vi "Drive Straight 2.vi"(9 "Time":dbl, 10 "Angle":dbl, 11 "RobotDriveDevRef in":T1) -> (3 "RobotDriveDevRef out":T1)   [LabVIEW 2015]
uses:
  <vilib>/Rock Robotics/WPI/RobotDrive/WPI_RobotDriveDevRef.ctl
  <vilib>/Rock Robotics/WPI/MotorControl/WPI_MotorControlDeviceRef.ctl
  <vilib>/Rock Robotics/WPI/MotorControl/WPI_MotorControlType.ctl
  <vilib>/Rock Robotics/SystemInterfaces/DIO/FPGA_DIOPWMChannel.ctl
  <vilib>/Rock Robotics/WPI/PWM/WPI_PWMDeadband.ctl
  <vilib>/Rock Robotics/WPI/CAN/Jaguar/SubVIs/WPI_CANJaguar_ControlMode.ctl
  <vilib>/Rock Robotics/WPI/CAN/TalonSRX/WPI_CANTalonSRX_APIControlMode.ctl
  <vilib>/Rock Robotics/Network Tables/NT Read Number.vi
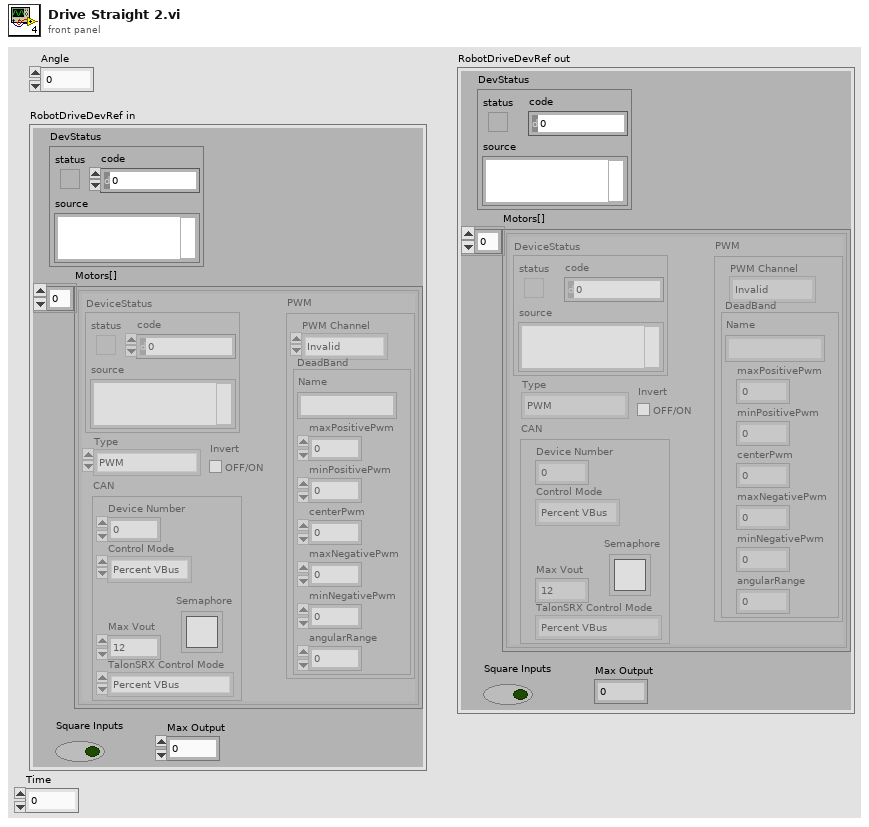
[diagram p1: front panel]
types:
  T1 = typedef "WPI_RobotDriveDevRef.ctl" = cluster{"DevStatus":errorcluster, "Motors[]":T2[], "Square Inputs":bool, "Max Output":dbl}
  T2 = typedef "WPI_MotorControlDeviceRef.ctl" = cluster{"DeviceStatus":errorcluster, "Type":T3, "PWM":cluster{"PWM Channel":T4, "DeadBand":T5}, "CAN":cluster{"Device Number":u8, "Control Mode":T6, "Semaphore":T7, "Max Vout":dbl, "TalonSRX Control Mode":T8}, "Invert":bool}
  T3 = typedef "WPI_MotorControlType.ctl" = enum16{"PWM", "CAN", "CANTalonSRX"}
  T4 = typedef "FPGA_DIOPWMChannel.ctl" = enum8{"PWM 0", "PWM 1", "PWM 2", "PWM 3", "PWM 4", "PWM 5", "PWM 6", "PWM 7", "PWM 8", "PWM 9", "PWM MXP 0", "PWM MXP 1", "PWM MXP 2", "PWM MXP 3", "PWM MXP 4", "PWM MXP 5", "PWM MXP 6", "PWM MXP 7", "PWM MXP 8", "PWM MXP 9", "Invalid"}
  T5 = typedef "WPI_PWMDeadband.ctl" = cluster{"Name":string, "maxPositivePwm":i32, "minPositivePwm":i32, "centerPwm":i32, "maxNegativePwm":i32, "minNegativePwm":i32, "angularRange":u16}
  T6 = typedef "WPI_CANJaguar_ControlMode.ctl" = enum8{"Percent VBus", "Current", "Speed", "Position", "Voltage"}
  T7 = typedef "Semaphore RefNum" = refnum<k1>
  T8 = typedef "WPI_CANTalonSRX_APIControlMode.ctl" = enum8{"Percent VBus", "Speed", "Position", "Slave", "Unchanged / Invalid", "Voltage Compensation", "Current", "Motion Profile"}
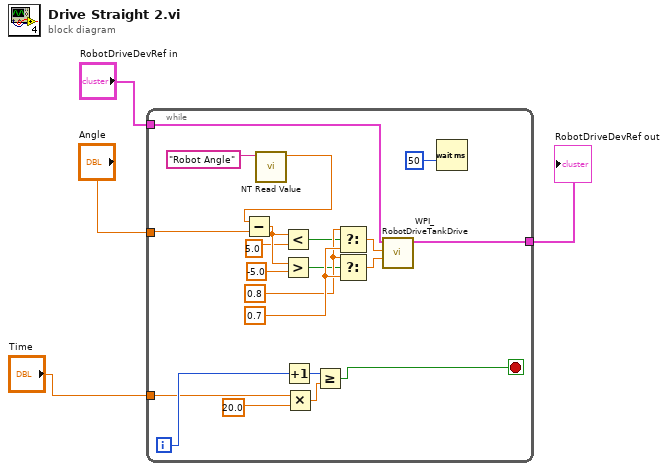
[diagram p0: block diagram]
diagram:
  n1 = while {
    tunnel: "Angle" -> [w20]
    tunnel: "RobotDriveDevRef in" -> [w18]
    tunnel: [w17] -> w2
    tunnel: "Time" -> [w6]
    i -> [w8]
    stop <- w7 stop-if-true
    w23 = 0.7
    w22 = 0.8
    n2 = call-poly <vilib>:"NT Read Value.vi"("Name"="Robot Angle") -> ("Numeric"=w21:dbl)  [unwired: 9 in, 1 out]
    n3 = Subtract(x=w21, y=w20) -> (x-y=w12:dbl)
    n4 = Less?(x=w12, y=5.0) -> (x < y?=w13:bool)
    n5 = Greater?(x=w12, y=-5.0) -> (0:w14:bool)
    n6 = Increment(x=w8) -> (x+1=w10:i32)
    n7 = Multiply(x=w6, y=20.0) -> (x*y=w9:dbl)
    n8 = Greater Or Equal?(x=w10, y=w9) -> (x >= y?=w7:bool)
    n9 = Select(t=w22, s=w13, f=w23) -> (s? t:f=w24:dbl)
    n10 = Select(t=w22, s=w14, f=w23) -> (s? t:f=w25:dbl)
    n11 = call <vilib>:"WPI_RobotDriveTankDrive.vi"("Right axis value"=w25, "Left axis value"=w24, "RobotDriveDevRef"=w18) -> ("RobotDriveDevRef"=w17:T1)  [unwired: 6 in, 2 out]
    n12 = Wait (ms)(milliseconds to wait=u32 50) -> ()  [unwired: 1 out]
  }
  "RobotDriveDevRef out" <- w2
